vi "runTestScenario.vi"(8 "error in (no error)":errorcluster, 11 "+5VDSupplyTest in":refnum<class "+5VDSupplyTest.lvclass">) -> (0 "error out":errorcluster, 2 "TestExecution":T1, 3 "+5VDSupplyTest out":refnum<class "+5VDSupplyTest.lvclass">)   [LabVIEW 2015, in "+5VDSupplyTest.lvclass"]
uses:
  +5VDSupplyTest.lvclass
  Typedefs/TestExecution.ctl
  Typedefs/WriteDataFileInput.ctl
  Typedefs/TestScenarioTypes.ctl
  Typedefs/WriteLogMessageInput.ctl
  Typedefs/PassFailTest.ctl
  +5VDSupplyTest.lvclass/+5VDSupplyTest.ctl
  Model/TestLog/ITestLog/ITestLog.lvclass
  Typedefs/ILCBTTypedefs.lvlib
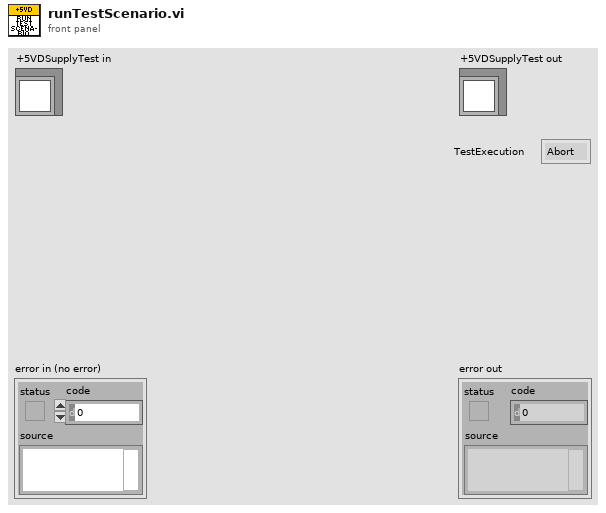
[diagram p1: front panel]
types:
  T1 = typedef "ILCBTTypedefs.lvlib/TestExecution.ctl" = enum16{"Abort", "Continue"}
  T2 = typedef "ILCBTTypedefs.lvlib/WriteLogMessageInput.ctl" = cluster{"Test Scenario":T3, "Description":string, "Actual Value":string, "Data File":string, "Result":T4}
  T3 = typedef "ILCBTTypedefs.lvlib/TestScenarioTypes.ctl" = enum16{"+3.3VA Supply Test", "+3.3VD Supply Test", "+5VA Supply Test", "+5VD Supply Test"}
  T4 = typedef "ILCBTTypedefs.lvlib/PassFailTest.ctl" = enum16{"Fail", "Pass", "NA"}
  T5 = typedef "ILCBTTypedefs.lvlib/WriteDataFileInput.ctl" = cluster{"Test Scenario":T3, "File Name":string, "Output":dbl[]}
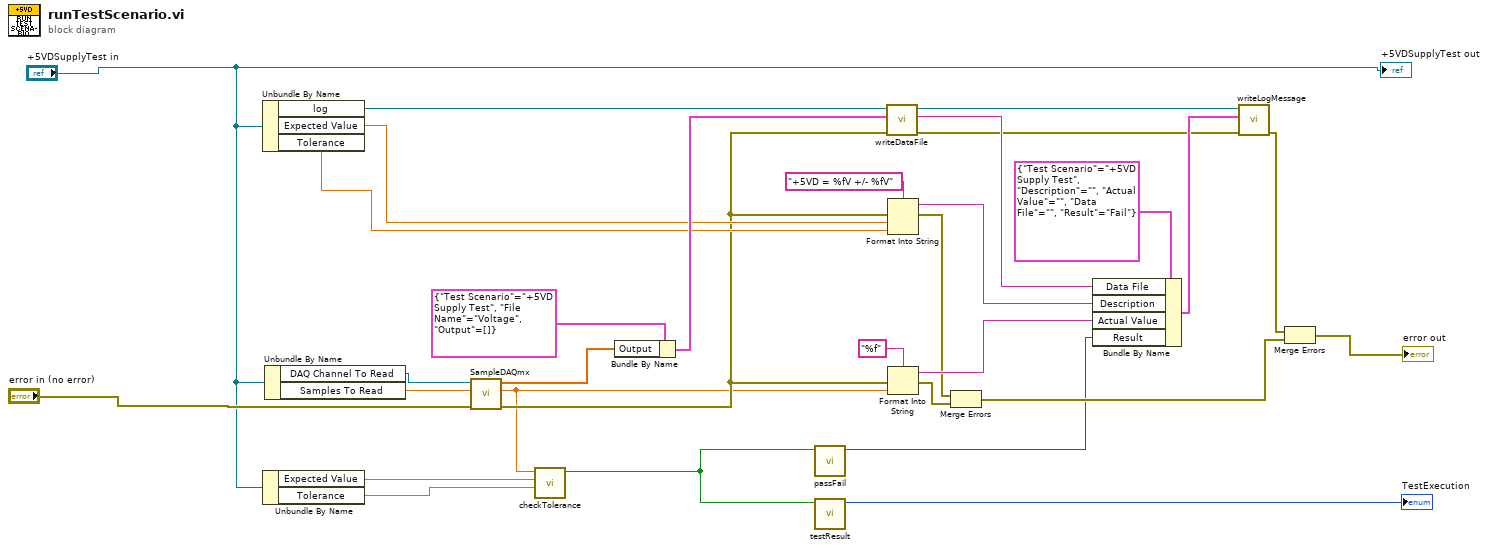
[diagram p0: block diagram]
diagram:
  n1 = Unbundle By Name("+5VDSupplyTest in") -> ("log"=w31:refnum<class "ITestLog.lvclass">, "Expected Value"=w20:dbl[unit], "Tolerance"=w19:dbl[unit])
  n2 = Unbundle By Name("+5VDSupplyTest in") -> ("Expected Value"=w3:dbl[unit], "Tolerance"=w2:dbl[unit])
  n3 = Unbundle By Name("+5VDSupplyTest in") -> ("DAQ Channel To Read"=w24:refnum<k21>, "Samples To Read"=w23:dbl)
  n4 = call "SampleDAQmx.vi"("error in (no error)"="error in (no error)", "Samples To Read"=w23, "DAQ Channel To Read"=w24) -> ("error out"=w18:errorcluster, "Average"=w4:dbl, "Samples"=w30:dbl[])  [unwired: 6 in]
  n5 = call "checkTolerance.vi"("Tolerance"=w2, "Expected Value"=w3, "Average"=w4) -> ("Boolean"=w1:bool)  [unwired: 8 in]
  n6 = Bundle By Name(cluster=T5 {"Test Scenario"=enum."+5VD Supply Test", "File Name"="Voltage", "Output"=[]} ("WriteDataFileInput"), "Output"=w30) -> (w21:T5)
  n7 = call "passFail.vi"("Boolean"=w1) -> ("Result"=w6:T4)  [unwired: 10 in]
  n8 = call "testResult.vi"("Boolean"=w1) -> ("TestExecution"=→"TestExecution":T1)  [unwired: 10 in]
  n9 = call-dynamic "writeDataFile.vi"("error in (no error)"=w18, "WriteDataFileInput"=w21, "ITestLog in"=w31) -> ("error out"=w14:errorcluster, "Relative Path"=w17:string, "ITestLog out"=w26:refnum<class "ITestLog.lvclass">)  [unwired: 6 in]
  n10 = Format Into String(format string="+5VD = %fV +/- %fV", error in=w18, w20, w19) -> (resulting string=w16:string, error out=w13:errorcluster)  [unwired: 1 in]
  n11 = Format Into String(format string="%f", error in=w18, w4) -> (resulting string=w15:string, error out=w12:errorcluster)  [unwired: 1 in]
  n12 = Merge Errors(w13, w12) -> (w10:errorcluster)
  n13 = Bundle By Name(cluster=T2 {"Test Scenario"=enum."+5VD Supply Test", "Description"="", "Actual Value"="", "Data File"="", "Result"=enum."Fail"} ("WriteLogMessageInput"), "Data File"=w17, "Description"=w16, "Actual Value"=w15, "Result"=w6) -> (w25:T2)
  n14 = call-dynamic "writeLogMessage.vi"("error in (no error)"=w14, "WriteLogMessageInput"=w25, "ITestLog in"=w26) -> ("error out"=w11:errorcluster)  [unwired: 7 in, 1 out]
  n15 = Merge Errors(w11, w10) -> (→"error out":errorcluster)
  "+5VDSupplyTest out" <- "+5VDSupplyTest in"
